vi "Get Image Delays.vi"(8 "error in (no error)":errorcluster, 10 "frames":u16, 11 "Simulated_Header in":refnum<class "Simulated_Header.lvclass">) -> (0 "error out":errorcluster, 3 "Simulated_Header out":refnum<class "Simulated_Header.lvclass">)   [LabVIEW 2018, in "Simulated_Header.lvclass"]
uses:
  Simulated_Header.lvclass
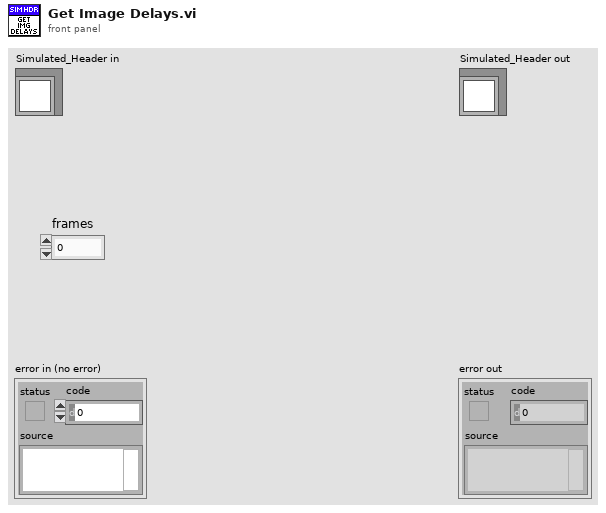
[diagram p1: front panel]
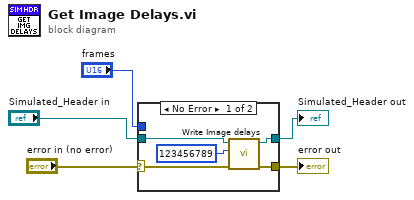
[diagram p0: block diagram]
diagram:
  n1 = case shown="No Error" "error in (no error)" {
    selector: "error in (no error)" -> [w9 w12]
    tunnel: [w7 w12] -> w3
    tunnel: [w8 w11] -> w2
    tunnel: "Simulated_Header in" -> [w10 w11]
    tunnel: "frames" -> [_ _]
    frame No Error {
      n2 = call "Write Image delays.vi"("error in (no error)"=w9, "Image Delays"=123456789, "Header in"=w10) -> ("error out"=w7:errorcluster, "Header out"=w8:refnum<class "Simulated_Header.lvclass">)  [unwired: 7 in]
    }
    frame Error {
    }
  }
  "error out" <- w3
  "Simulated_Header out" <- w2
